vi "q5 search and replace.vi"() -> ()   [LabVIEW 2025]
panel:
  out "result string":string
  in  "replacement":string
  in  "search":string
  in  "source":string
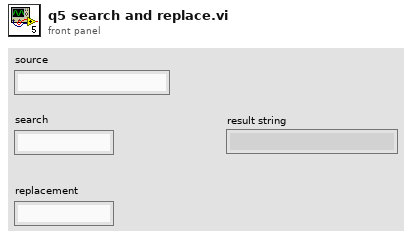
[diagram p1: front panel]
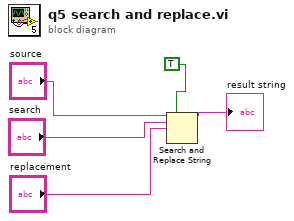
[diagram p0: block diagram]
diagram:
  n1 = Search and Replace String(replace all?=TRUE, input string="source", search string="search", replace string="replacement") -> (result string=→"result string":string)  [unwired: 4 in, 3 out]
